vi "x_h_dir_string.vi"(4 "xback":bool, 6 "xfwd":bool, 8 "hdown":bool, 9 "hup":bool, 10 "xdown":bool, 11 "xup":bool) -> (3 "x_h_dir":string)   [LabVIEW 2012]
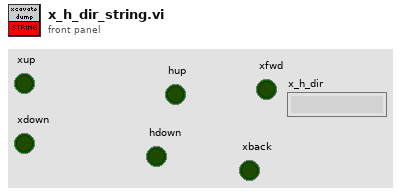
[diagram p1: front panel]
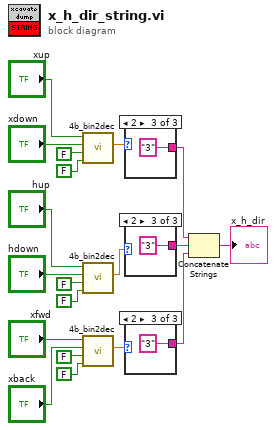
[diagram p0: block diagram]
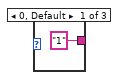
[diagram p2: hidden frame]
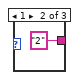
[diagram p3: hidden frame]
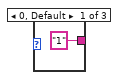
[diagram p4: hidden frame]
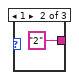
[diagram p5: hidden frame]
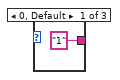
[diagram p6: hidden frame]
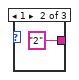
[diagram p7: hidden frame]
diagram:
  n1 = call "4b_bin2dec.vi"("Right"=FALSE, "Left"=FALSE, "Down"="xdown", "Up"="xup") -> ("Out"=w7:dbl)  [unwired: 7 in]
  n2 = call "4b_bin2dec.vi"("Right"=FALSE, "Left"=FALSE, "Down"="hdown", "Up"="hup") -> ("Out"=w6:dbl)  [unwired: 7 in]
  n3 = call "4b_bin2dec.vi"("Right"=FALSE, "Left"=FALSE, "Down"="xback", "Up"="xfwd") -> ("Out"=w5:dbl)  [unwired: 7 in]
  n4 = case shown="2" w7 {
    tunnel: ["1" "2" "3"] -> w4
    frame 0, Default {
    }
    frame 1 {
    }
    frame 2 {
    }
  }
  n5 = case shown="2" w6 {
    tunnel: ["1" "2" "3"] -> w3
    frame 0, Default {
    }
    frame 1 {
    }
    frame 2 {
    }
  }
  n6 = case shown="2" w5 {
    tunnel: ["1" "2" "3"] -> w2
    frame 0, Default {
    }
    frame 1 {
    }
    frame 2 {
    }
  }
  n7 = Concatenate Strings(w4, w3, w2) -> (→"x_h_dir":string)
